vi "LoadAutoReArm(mSec).vi"(8 "error in (no error)":errorcluster, 11 "TrigBoxINIFileClass in":refnum<class "TrigBoxINIFileClass.lvclass">) -> (0 "error out":errorcluster, 2 "AutoReArm(mSec)":i64, 3 "TrigBoxINIFileClass out":refnum<class "TrigBoxINIFileClass.lvclass">)   [LabVIEW 2013, in "TrigBoxINIFileClass.lvclass"]
uses:
  TrigBoxINIFileClass.lvclass
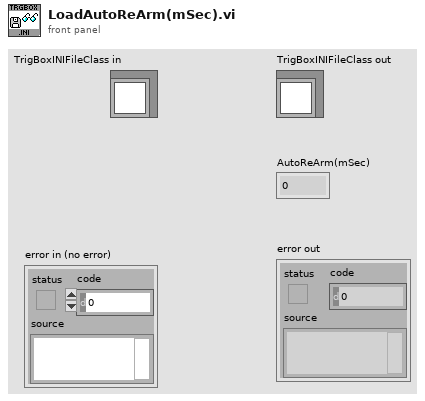
[diagram p1: front panel]
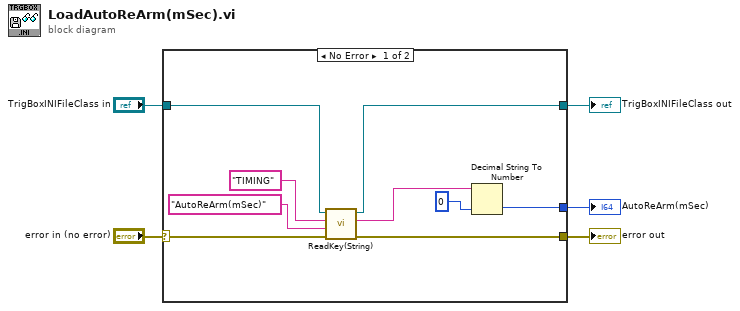
[diagram p0: block diagram]
diagram:
  n1 = case shown="No Error" "error in (no error)" {
    selector: "error in (no error)" -> [w12 w16]
    tunnel: [w6 w16] -> w4
    tunnel: [w8 w15] -> w2
    tunnel: "TrigBoxINIFileClass in" -> [w9 w15]
    tunnel: [w13 _] -> w1
    frame No Error {
      n2 = call-dynamic "ReadKey(String).vi"("error in"=w12, "key"="AutoReArm(mSec)" ("section"), "section"="TIMING", "INIFileClass in"=w9) -> ("error out"=w6:errorcluster, "StringOut"=w7:string, "INIFileClass out"=w8:refnum<class "TrigBoxINIFileClass.lvclass">)  [unwired: 5 in]
      n3 = Decimal String To Number(string=w7, default (0L)=i64 0) -> (number=w13:i64)  [unwired: 1 in, 1 out]
    }
    frame Error {
    }
  }
  "error out" <- w4
  "TrigBoxINIFileClass out" <- w2
  "AutoReArm(mSec)" <- w1
